vi "Name.vi"(8 "error in (no error)":errorcluster, 11 "Task in":refnum<class "Task.lvclass">) -> (0 "error out":errorcluster, 2 "Name":string, 3 "Task out":refnum<class "Task.lvclass">)   [LabVIEW 2020, in "VolatusConfig.lvlib" / "Task.lvclass"]
uses:
  Task.lvclass
  Task.lvclass/Task.ctl
  lv-cdm/CDM-Config/Config Element/Config Element.lvclass
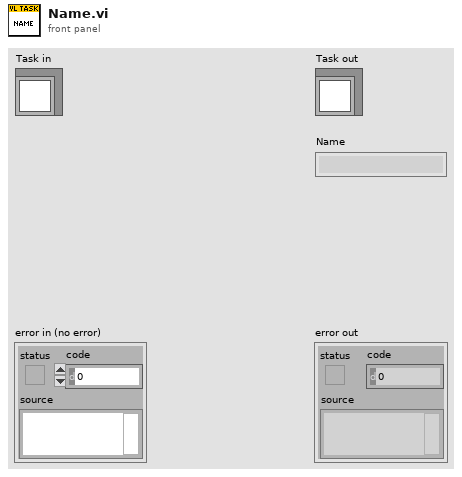
[diagram p1: front panel]
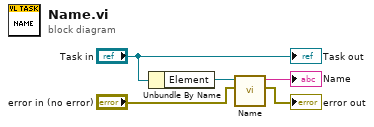
[diagram p0: block diagram]
diagram:
  n1 = Unbundle By Name("Task in") -> ("Element"=w4:refnum<class "Config Element.lvclass">)
  n2 = call "Name.vi"("error in (no error)"="error in (no error)", "Config Element in"=w4) -> ("error out"=→"error out":errorcluster, "Name"=→"Name":string)  [unwired: 8 in]
  "Task out" <- "Task in"
